vi "SPARK Set Parameter Int32.vi"(7 "Ignore":bool, 8 "error in (no error)":errorcluster, 9 "int":i32, 10 "Parameter ID":T6, 11 "MotorControlDeviceRef":T1={"DeviceStatus"={"status"=FALSE, "code"=0, "source"=""}, "Type"=enum."CAN", "PWM"={"PWM Channel"=enum."Invalid", "DeadBand"={"Name"="", "maxPositivePwm"=0, "minPositivePwm"=0, "centerPwm"=0, "maxNegativePwm"=0, "minNegativePwm"=0, "angularRange"=0}}, "CAN"={"Device Number"=8, "SetOutput VI Ref"=variant, "GetOutput VI Ref"=variant, "Enable VI Ref"=variant, "Disable VI Ref"=variant, "Data"=variant(cluster{"Ext ID":u32, "Motor Type":enum16{"Brushed", "Brushless"}} {"Ext ID"=33882120, "Motor Type"=enum."Brushed"})}, "Invert"=FALSE, "DIO PWM"={"PWM \"Enable\" Channel"=enum."Invalid", "DIOChannel"=enum."Invalid", "PWM Rate"=0.0}}) -> (0 "error out":errorcluster, 3 "MotorControlDeviceRef":T1={"DeviceStatus"={"status"=FALSE, "code"=0, "source"=""}, "Type"=enum."CAN", "PWM"={"PWM Channel"=enum."Invalid", "DeadBand"={"Name"="", "maxPositivePwm"=0, "minPositivePwm"=0, "centerPwm"=0, "maxNegativePwm"=0, "minNegativePwm"=0, "angularRange"=0}}, "CAN"={"Device Number"=8, "SetOutput VI Ref"=variant, "GetOutput VI Ref"=variant, "Enable VI Ref"=variant, "Disable VI Ref"=variant, "Data"=variant(cluster{"Ext ID":u32, "Motor Type":enum16{"Brushed", "Brushless"}} {"Ext ID"=33882120, "Motor Type"=enum."Brushed"})}, "Invert"=FALSE, "DIO PWM"={"PWM \"Enable\" Channel"=enum."Invalid", "DIOChannel"=enum."Invalid", "PWM Rate"=0.0}})   [LabVIEW 2023]
uses:
  Typedef/SPARK Parameter ID.ctl
  <vilib>/Rock Robotics/WPI/MotorControl/WPI_MotorControlDeviceRef.ctl
  <vilib>/Rock Robotics/WPI/MotorControl/WPI_MotorControlType.ctl
  <vilib>/Rock Robotics/SystemInterfaces/DIO/FPGA_DIOPWMChannel.ctl
  <vilib>/Rock Robotics/WPI/PWM/WPI_PWMDeadband.ctl
  <vilib>/Rock Robotics/SystemInterfaces/DIO/FPGA_DIOChannel.ctl
  9c35adcf-d745-4de8-910c-405e8d350018.vi
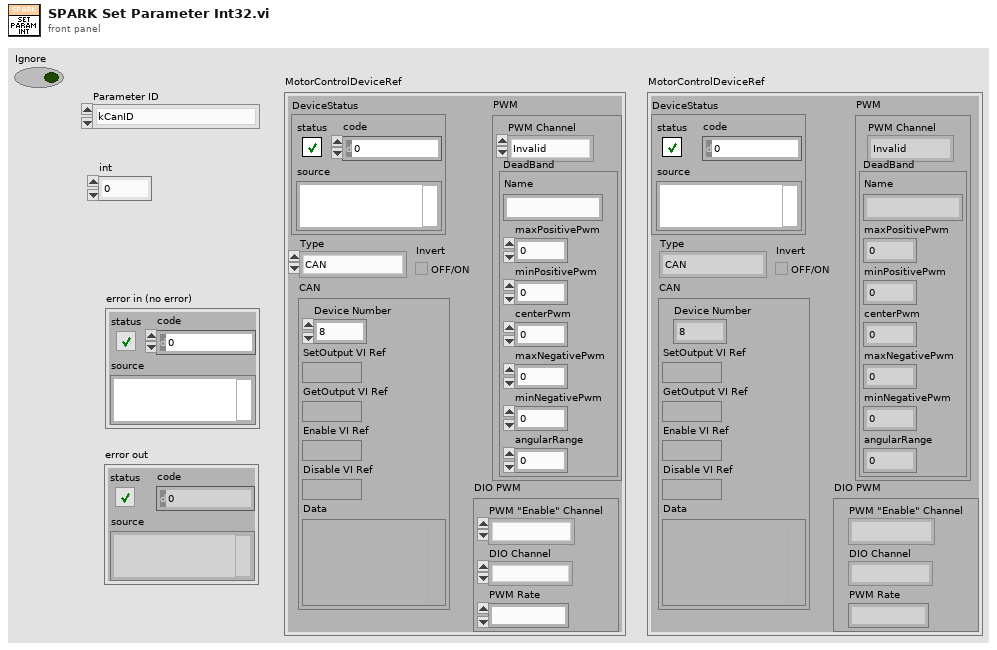
[diagram p1: front panel]
types:
  T1 = typedef "WPI_MotorControlDeviceRef.ctl" = cluster{"DeviceStatus":errorcluster, "Type":T2, "PWM":cluster{"PWM Channel":T3, "DeadBand":T4}, "CAN":cluster{"Device Number":u8, "SetOutput VI Ref":variant, "GetOutput VI Ref":variant, "Enable VI Ref":variant, "Disable VI Ref":variant, "Data":variant}, "Invert":bool, "DIO PWM":cluster{"PWM \"Enable\" Channel":T3, "DIOChannel":T5, "PWM Rate":dbl}}
  T2 = typedef "WPI_MotorControlType.ctl" = enum16{"PWM", "CAN", "DIO PWM"}
  T3 = typedef "FPGA_DIOPWMChannel.ctl" = enum8{"PWM 0", "PWM 1", "PWM 2", "PWM 3", "PWM 4", "PWM 5", "PWM 6", "PWM 7", "PWM 8", "PWM 9", "PWM MXP 0", "PWM MXP 1", "PWM MXP 2", "PWM MXP 3", "PWM MXP 4", "PWM MXP 5", "PWM MXP 6", "PWM MXP 7", "PWM MXP 8", "PWM MXP 9", "Invalid"}
  T4 = typedef "WPI_PWMDeadband.ctl" = cluster{"Name":string, "maxPositivePwm":i32, "minPositivePwm":i32, "centerPwm":i32, "maxNegativePwm":i32, "minNegativePwm":i32, "angularRange":u16}
  T5 = typedef "FPGA_DIOChannel.ctl" = enum8{"DIO 0", "DIO 1", "DIO 2", "DIO 3", "DIO 4", "DIO 5", "DIO 6", "DIO 7", "DIO 8", "DIO 9", "DIO MXP 0", "DIO MXP 1", "DIO MXP 2", "DIO MXP 3", "DIO MXP 4", "DIO MXP 5", "DIO MXP 6", "DIO MXP 7", "DIO MXP 8", "DIO MXP 9", "DIO MXP 10", "DIO MXP 11", "DIO MXP 12", "DIO MXP 13", "DIO MXP 14", "DIO MXP 15", "SPI Port CS1", "SPI Port CS2", "SPI Port CS3", "SPI Port MISO", "SPI Port MOSI", "Invalid"}
  T6 = typedef "SPARK Parameter ID.ctl" = enum16{"kCanID", "kInputMode", "kMotorType", "kCommAdvance", "kSensorType", "kCtrlType", "kIdleMode", "kInputDeadband", "kLegacyFeedbackSensorPID0", "kClosedLoopControlSensor", "kPolePairs", "kCurrentChop", "kCurrentChopCycles", "kP_0", "kI_0", "kD_0", "kF_0", "kIZone_0", "kDFilter_0", "kOutputMin_0", "kOutputMax_0", "kP_1", "kI_1", "kD_1", "kF_1", "kIZone_1", "kDFilter_1", "kOutputMin_1", "kOutputMax_1", "kP_2", "kI_2", "kD_2", "kF_2", "kIZone_2", "kDFilter_2", "kOutputMin_2", "kOutputMax_2", "kP_3", "kI_3", "kD_3", "kF_3", "kIZone_3", "kDFilter_3", "kOutputMin_3", "kOutputMax_3", "kInverted", "kOutputRatio", "kSerialNumberLow", "kSerialNumberMid", "kSerialNumberHigh", "kLimitSwitchFwdPolarity", "kLimitSwitchRevPolarity", "kHardLimitFwdEn", "kHardLimitRevEn", "kSoftLimitFwdEn", "kSoftLimitRevEn", "kRampRate", "kFollowerID", "kFollowerConfig", "kSmartCurrentStallLimit", "kSmartCurrentFreeLimit", "kSmartCurrentConfig", "kSmartCurrentReserved", "kMotorKv", "kMotorR", "kMotorL", "kMotorRsvd1", "kMotorRsvd2", "kMotorRsvd3", "kEncoderCountsPerRev", "kEncoderAverageDepth", "kEncoderSampleDelta", "kEncoderInverted", "kEncoderRsvd1", "kClosedLoopVoltageMode", "kCompensatedNominalVoltage", "kSmartMotionMaxVelocity_0", "kSmartMotionMaxAccel_0", "kSmartMotionMinVelOutput_0", "kSmartMotionAllowedClosedLoopError_0", "kSmartMotionAccelStrategy_0", "kSmartMotionMaxVelocity_1", "kSmartMotionMaxAccel_1", "kSmartMotionMinVelOutput_1", "kSmartMotionAllowedClosedLoopError_1", "kSmartMotionAccelStrategy_1", "kSmartMotionMaxVelocity_2", "kSmartMotionMaxAccel_2", "kSmartMotionMinVelOutput_2", "kSmartMotionAllowedClosedLoopError_2", "kSmartMotionAccelStrategy_2", "kSmartMotionMaxVelocity_3", "kSmartMotionMaxAccel_3", "kSmartMotionMinVelOutput_3", "kSmartMotionAllowedClosedLoopError_3", "kSmartMotionAccelStrategy_3", "kIMaxAccum_0", "kSlot3Placeholder1_0", "kSlot3Placeholder2_0", "kSlot3Placeholder3_0", "kIMaxAccum_1", "kSlot3Placeholder1_1", "kSlot3Placeholder2_1", "kSlot3Placeholder3_1", "kIMaxAccum_2", "kSlot3Placeholder1_2", "kSlot3Placeholder2_2", "kSlot3Placeholder3_2", "kIMaxAccum_3", "kSlot3Placeholder1_3", "kSlot3Placeholder2_3", "kSlot3Placeholder3_3", "kPositionConversionFactor", "kVelocityConversionFactor", "kClosedLoopRampRate", "kSoftLimitFwd", "kSoftLimitRev", "kSoftLimitRsvd0", "kSoftLimitRsvd1", "kAnalogPositionConversion", "kAnalogVelocityConversion", "kAnalogAverageDepth", "kAnalogSensorMode", "kAnalogInverted", "kAnalogSampleDelta", "kAnalogRsvd0", "kAnalogRsvd1", "kDataPortConfig", "kAltEncoderCountsPerRev", "kAltEncoderAverageDepth", "kAltEncoderSampleDelta", "kAltEncoderInverted", "kAltEncoderPositionConversion", "kAltEncoderVelocityConversion", "kAltEncoderRsvd0", "kAltEncoderRsvd1", "kHallSensorSampleRate", "kHallSensorAverageDepth", "kNumParameters", "kDutyCyclePositionFactor", "kDutyCycleVelocityFactor", "kDutyCycleInverted", "kDutyCycleSensorMode", "kDutyCycleAverageDepth", "kDutyCycleSampleDelta", "kDutyCycleOffsetv1p6p2", "kDutyCycleRsvd0", "kDutyCycleRsvd1", "kDutyCycleRsvd2", "kPositionPIDWrapEnable", "kPositionPIDMinInput", "kPositionPIDMaxInput", "kDutyCycleZeroCentered", "kDutyCyclePrescalar", "kDutyCycleOffset", "kProductId", "kDeviceMajorVersion", "kDeviceMinorVersion", "kStatus0Period", "kStatus1Period", "kStatus2Period", "kStatus3Period", "kStatus4Period", "kStatus5Period", "kStatus6Period", "kStatus7Period", "kMAXMotionMaxVelocity_0", "kMAXMotionMaxAccel_0", "kMAXMotionMaxJerk_0", "kMAXMotionAllowedClosedLoopError_0", "kMAXMotionPositionMode_0", "kMAXMotionMaxVelocity_1", "kMAXMotionMaxAccel_1", "kMAXMotionMaxJerk_1", "kMAXMotionAllowedClosedLoopError_1", "kMAXMotionPositionMode_1", "kMAXMotionMaxVelocity_2", "kMAXMotionMaxAccel_2", "kMAXMotionMaxJerk_2", "kMAXMotionAllowedClosedLoopError_2", "kMAXMotionPositionMode_2", "kMAXMotionMaxVelocity_3", "kMAXMotionMaxAccel_3", "kMAXMotionMaxJerk_3", "kMAXMotionAllowedClosedLoopError_3", "kMAXMotionPositionMode_3", "kForceEnableStatus0", "kForceEnableStatus1", "kForceEnableStatus2", "kForceEnableStatus3", "kForceEnableStatus4", "kForceEnableStatus5", "kForceEnableStatus6", "kForceEnableStatus7", "kFollowerModeLeaderId", "kFollowerModeIsInverted", "kDutyCycleEncoderStartPulseUs", "kDutyCycleEncoderEndPulseUs"}
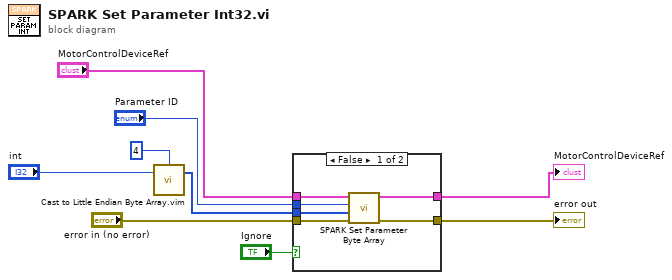
[diagram p0: block diagram]
diagram:
  n1 = call "Cast to Little Endian Byte Array.vim"("value"="int", "bytes"=4 ("dimension size (4)")) -> ("output array"=w6:u8[])  [unwired: 1 in]
  n2 = case shown="False" "Ignore" {
    tunnel: "MotorControlDeviceRef" -> [w15 w17]
    tunnel: w6 -> [w14 _]
    tunnel: "Parameter ID" -> [w13 _]
    tunnel: [w12 w16] -> w4
    tunnel: "error in (no error)" -> [w11 w16]
    tunnel: [w10 w17] -> w2
    frame False {
      n3 = call "SPARK Set Parameter Byte Array.vi"("error in (no error)"=w11, "Bytes LSB First"=w14, "Parameter ID"=w13, "MotorControlDeviceRef"=w15) -> ("error out"=w12:errorcluster, "MotorControlDeviceRef"=w10:T1)  [unwired: 6 in]
    }
    frame True {
    }
  }
  "error out" <- w4
  "MotorControlDeviceRef" <- w2
